vi "LED.vi"() -> ()   [LabVIEW 2018]
panel:
  in  "Boolean":bool
  out "x-y*floor(x/y)":i32
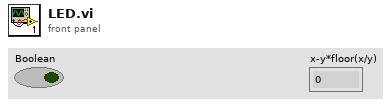
[diagram p1: front panel]
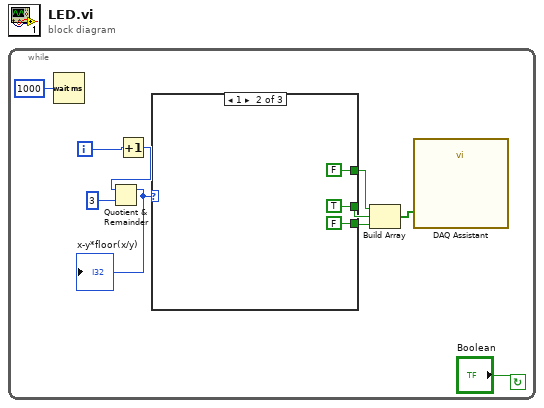
[diagram p0: block diagram]
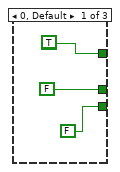
[diagram p2: hidden frame]
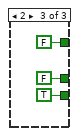
[diagram p3: hidden frame]
diagram:
  n1 = while {
    i -> [w8]
    stop <- "Boolean" continue-if-true
    n2 = Wait (ms)(milliseconds to wait=u32 1000) -> ()  [unwired: 1 out]
    n3 = Increment(x=w8) -> (x+1=w9:i32)
    n4 = Quotient & Remainder(x=w9, y=3) -> (x-y*floor(x/y)=w10:i32)  [unwired: 1 out]
    "x-y*floor(x/y)" <- w10
    n5 = case shown="1" w10 {
      tunnel: [FALSE FALSE TRUE] -> w5
      tunnel: [FALSE TRUE FALSE] -> w3
      tunnel: [TRUE FALSE FALSE] -> w4
      frame 0, Default {
        (unwired) TRUE
      }
      frame 1 {
      }
      frame 2 {
      }
    }
    n6 = Build Array(w4, w3, w5) -> (w2:bool[])
    n7 = call "DAQ Assistant"("data"=w2) -> ()  [unwired: 17 in, 2 out]
  }
